vi "Read Inserted VI.vi"(8 "error in (no error)":errorcluster, 11 "GetSubPanelVI in":refnum<class "GetSubPanelVI.lvclass">) -> (0 "error out":errorcluster, 2 "Inserted VI":refnum<vi>, 3 "GetSubPanelVI out":refnum<class "GetSubPanelVI.lvclass">)   [LabVIEW 2016, in "GetSubPanelVI.lvclass"]
uses:
  GetSubPanelVI.lvclass
  GetSubPanelVI.lvclass/GetSubPanelVI.ctl
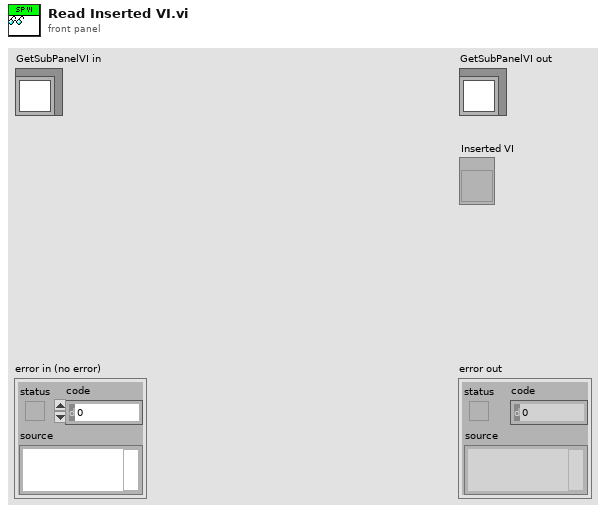
[diagram p1: front panel]
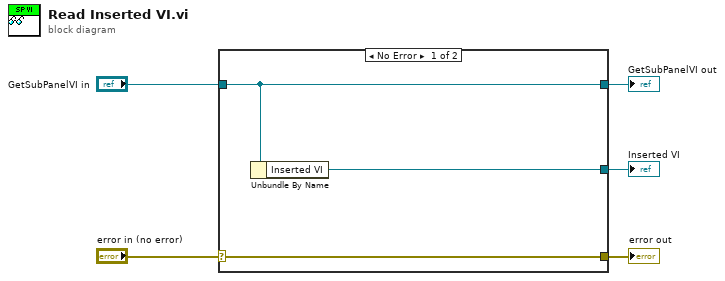
[diagram p0: block diagram]
diagram:
  n1 = case shown="No Error" "error in (no error)" {
    selector: "error in (no error)" -> [w8 w9]
    tunnel: [w8 w9] -> w4
    tunnel: [w7 w10] -> w2
    tunnel: "GetSubPanelVI in" -> [w7 w10]
    tunnel: [w6 _] -> w1
    frame No Error {
      n2 = Unbundle By Name(w7) -> ("Inserted VI"=w6:refnum<vi>)
    }
    frame Error {
    }
  }
  "error out" <- w4
  "GetSubPanelVI out" <- w2
  "Inserted VI" <- w1
